vi "Get FPGA Name From Monkey ID.vi"(8 "error in (no error)":errorcluster, 10 "Monkey ID":string, 11 "Tamer in":refnum<class "Tamer.lvclass">) -> (0 "error out":errorcluster, 2 "FPGA Name":string, 3 "Tamer out":refnum<class "Tamer.lvclass">)   [LabVIEW 2020, in "Tamer.lvlib" / "Tamer.lvclass"]
uses:
  Tamer.lvclass
  Tamer.lvclass/Tamer.ctl
  TALOS/TALOS_PPL.lvlibp
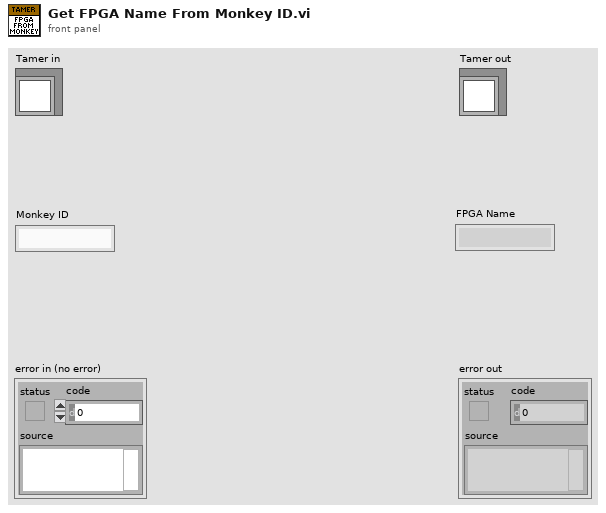
[diagram p1: front panel]
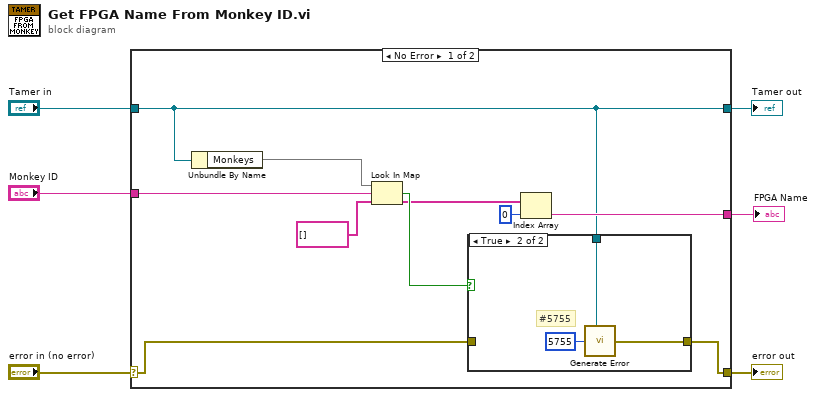
[diagram p0: block diagram]
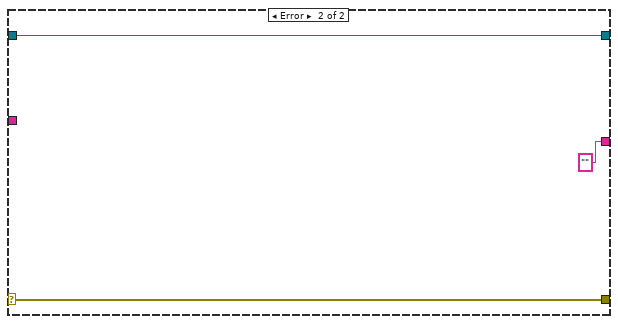
[diagram p3: hidden frame]
diagram:
  n1 = case shown="No Error" "error in (no error)" {
    selector: "error in (no error)" -> [w12 w23]
    tunnel: [w7 w23] -> w5
    tunnel: [w8 w22] -> w3
    tunnel: "Tamer in" -> [w8 w22]
    tunnel: "Monkey ID" -> [w15 _]
    tunnel: [w10 "" ("Kasli Name")] -> w1
    frame No Error {
      n2 = Unbundle By Name(w8) -> ("Monkeys"=w16:map{string, string[]})
      n3 = Look In Map(map=w16, key=w15, default value=string[] []) -> (key not found?=w13:bool, value=w11:string[])
      n4 = case shown="True" w13 {
        tunnel: w12 -> [w17 _]
        tunnel: w8 -> [_ w20]
        tunnel: [w17 w19] -> w7
        frame False {
        }
        frame True {
          # "#5755"
          n5 = call "Generate Error.vi"("Class"=w20, "Error Code"=5755) -> ("error out"=w19:errorcluster)  [unwired: 5 in]
        }
      }
      n6 = Index Array(array=w11, index=0) -> (element=w10:string)
    }
    frame Error {
    }
  }
  "error out" <- w5
  "Tamer out" <- w3
  "FPGA Name" <- w1
